vi "Get Name.vi"(8 "error in (no error)":errorcluster, 11 "Device in":refnum<class "Device.lvclass">) -> (0 "error out":errorcluster, 2 "Name":string, 3 "Device out":refnum<class "Device.lvclass">)   [LabVIEW 2012, in "HAL.lvlib" / "Device.lvclass"]
uses:
  Device.lvclass
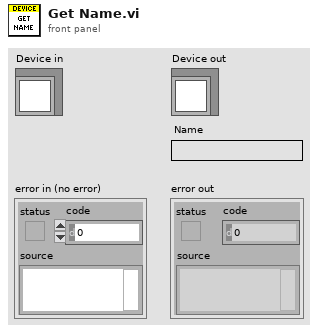
[diagram p1: front panel]
types:
  T1 = typedef "HAL.lvlib/Device.lvclass/Ref Data.ctl" = cluster{"Config Keys":string[], "Config Values":string[], "Cal Expires":timestamp, "Name":string, "Comment":string, "State":T2, "Error":errorcluster}
  T2 = typedef "HAL.lvlib/Device.lvclass/Device State.ctl" = enum16{"Uninitialized", "Initialized", "Ready", "Running", "Error"}
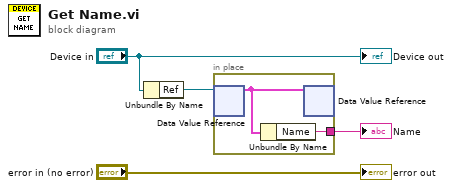
[diagram p0: block diagram]
diagram:
  n1 = Unbundle By Name("Device in") -> ("Ref"=w3:refnum<data-value>)
  n2 = in-place {
    in-place-border: [w5] -> w1
    n3 = in-place-dvr #1(w3) -> (w6:T1)  [unwired: 1 out]
    n4 = Unbundle By Name(w6) -> ("Name"=w5:string)
    n5 = in-place-dvr #1(w6) -> ()  [unwired: 2 out]
  }
  "Name" <- w1
  "error out" <- "error in (no error)"
  "Device out" <- "Device in"
